vi "Add_TestReportFolder.vi"(8 "error in (no error)":errorcluster caption="错误输入（无错误）", 10 "是否新建多类文件夹":bool, 11 "path":path) -> (0 "错误输出":errorcluster, 1 "XLM path":path, 2 "TXT path":path, 3 "CSV path":path, 5 "Log path":path)   [LabVIEW 2018]
panel:
  out "EXCLE path":path
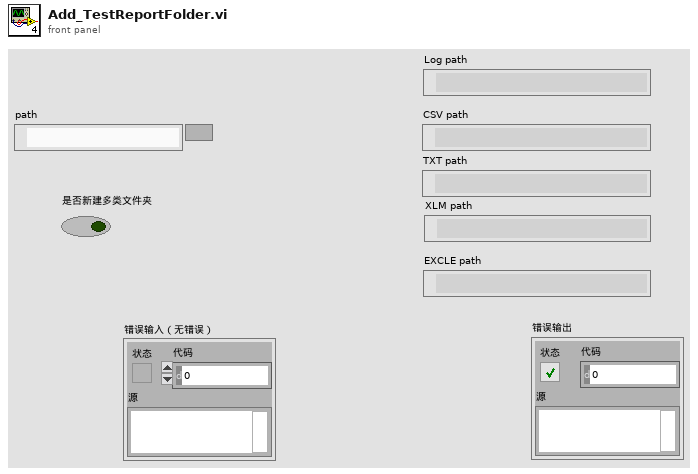
[diagram p1: front panel]
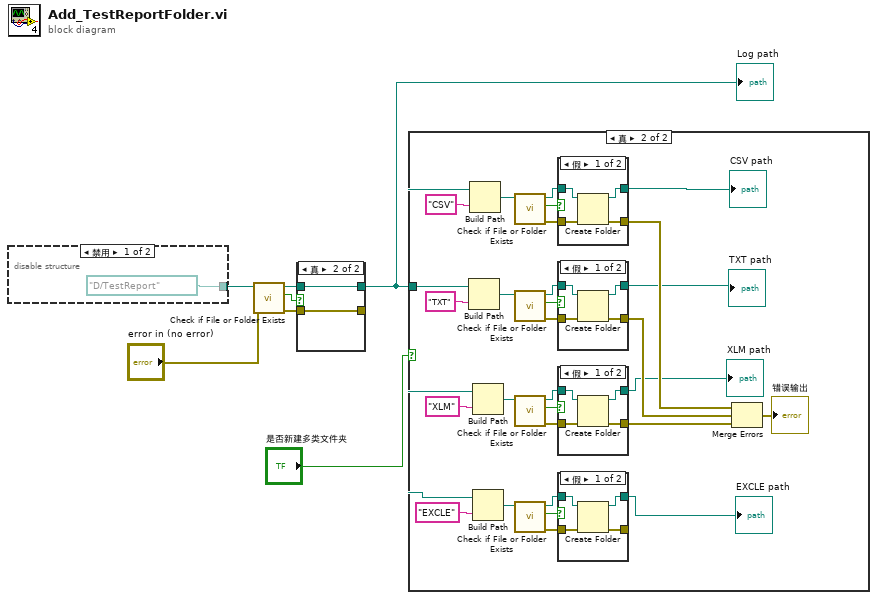
[diagram p0: block diagram]
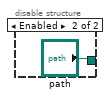
[diagram p7: hidden frame]
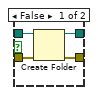
[diagram p8: hidden frame]
diagram:
  n1 = disable-structure shown="禁用" {
    disable-tunnel: [path "D:/TestReport" ("path") "path"] -> w7
    frame Disabled {
    }
    frame Enabled {
    }
  }
  n2 = call <vilib>:"Check if File or Folder Exists.vi"("error in (no error)"="error in (no error)", "path"=w7) -> ("error out"=w4:errorcluster, "file or folder exists?"=w5:bool, "dup path"=w6:path)  [unwired: 7 in]
  n3 = case shown="真" w5 {
    tunnel: w6 -> [w13 w15]
    tunnel: [w12 w15] -> w2
    tunnel: w4 -> [w11 w14]
    tunnel: [w10 w14] -> _
    frame False {
      n4 = Create Folder(path (use dialog)=w13, error in=w11) -> (created path=w12:path, error out=w10:errorcluster)  [unwired: 1 in, 1 out]
    }
    frame True {
    }
  }
  "Log path" <- w2
  n5 = case shown="真" "是否新建多类文件夹" {
    tunnel: w2 -> [_ w16]
    frame False {
    }
    frame True {
      n6 = Build Path(base path=w16, name or relative path="TXT" ("名称或相对路径")) -> (appended path=w33:path)
      n7 = Build Path(base path=w16, name or relative path="CSV" ("名称或相对路径")) -> (appended path=w39:path)
      n8 = Build Path(base path=w16, name or relative path="XLM" ("名称或相对路径")) -> (appended path=w34:path)
      n9 = Build Path(base path=w16, name or relative path="EXCLE" ("名称或相对路径")) -> (appended path=w20:path)
      n10 = call <vilib>:"Check if File or Folder Exists.vi"("path"=w39) -> ("error out"=w28:errorcluster, "file or folder exists?"=w41:bool, "dup path"=w40:path)  [unwired: 8 in]
      n11 = call <vilib>:"Check if File or Folder Exists.vi"("path"=w33) -> ("error out"=w29:errorcluster, "file or folder exists?"=w37:bool, "dup path"=w38:path)  [unwired: 8 in]
      n12 = call <vilib>:"Check if File or Folder Exists.vi"("path"=w34) -> ("error out"=w31:errorcluster, "file or folder exists?"=w36:bool, "dup path"=w35:path)  [unwired: 8 in]
      n13 = call <vilib>:"Check if File or Folder Exists.vi"("path"=w20) -> ("error out"=w21:errorcluster, "file or folder exists?"=w18:bool, "dup path"=w19:path)  [unwired: 8 in]
      n14 = case shown="假" w41 {
        tunnel: w40 -> [w66 w68]
        tunnel: [w65 w68] -> w25
        tunnel: w28 -> [w64 w67]
        tunnel: [w63 w67] -> w27
        frame False {
          n15 = Create Folder(path (use dialog)=w66, error in=w64) -> (created path=w65:path, error out=w63:errorcluster)  [unwired: 1 in, 1 out]
        }
        frame True {
        }
      }
      "CSV path" <- w25
      n16 = case shown="假" w37 {
        tunnel: w38 -> [w60 w62]
        tunnel: [w59 w62] -> w24
        tunnel: [w58 w61] -> w30
        tunnel: w29 -> [w57 w61]
        frame False {
          n17 = Create Folder(path (use dialog)=w60, error in=w57) -> (created path=w59:path, error out=w58:errorcluster)  [unwired: 1 in, 1 out]
        }
        frame True {
        }
      }
      "TXT path" <- w24
      n18 = case shown="假" w36 {
        tunnel: w35 -> [w54 w56]
        tunnel: [w53 w56] -> w23
        tunnel: [w52 w55] -> w32
        tunnel: w31 -> [w51 w55]
        frame False {
          n19 = Create Folder(path (use dialog)=w54, error in=w51) -> (created path=w53:path, error out=w52:errorcluster)  [unwired: 1 in, 1 out]
        }
        frame True {
        }
      }
      "XLM path" <- w23
      n20 = case shown="假" w18 {
        tunnel: w19 -> [w48 w50]
        tunnel: [w47 w50] -> w22
        tunnel: [w46 w49] -> _
        tunnel: w21 -> [w45 w49]
        frame False {
          n21 = Create Folder(path (use dialog)=w48, error in=w45) -> (created path=w47:path, error out=w46:errorcluster)  [unwired: 1 in, 1 out]
        }
        frame True {
        }
      }
      "EXCLE path" <- w22
      n22 = Merge Errors(w27, w30, w32) -> (→"错误输出":errorcluster)
    }
  }
